vi "(Depricated) Sample Trasfer Base Pressure Mean.vi"(3 "sample length (10)":i32=10, 4 "initialize on the next call":bool, 5 "Baratron 1":dbl format="%0.2f") -> (0 "d":dbl(graph), 1 "mean":dbl format="%0.2f")   [LabVIEW 2015, in "cRIO-Carbondioxide.lvlib" / "cRIO-CO2.lvlib" / "cRIO-CO2.lvclass"]
uses:
  cRIO-CO2.lvclass
  <vilib>/ptbypt/NI_PtbyPt.lvlib
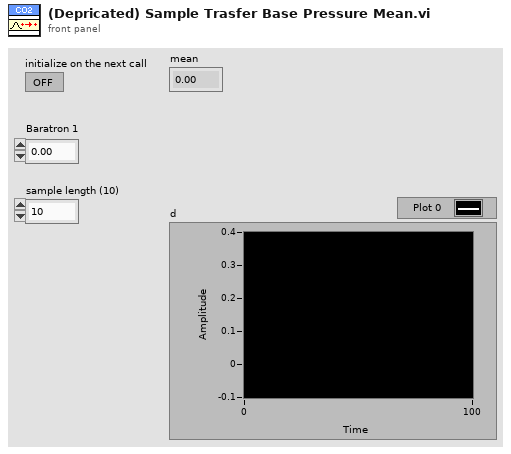
[diagram p1: front panel]
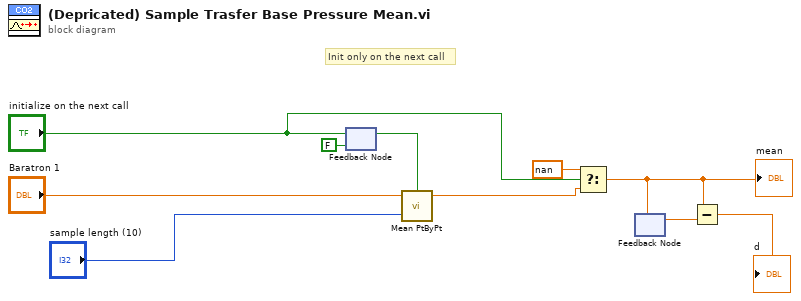
[diagram p0: block diagram]
diagram:
  # "Init only on the next call"
  n1 = feedback-in #1("initialize on the next call") -> ()
  n2 = feedback #1(FALSE ("initialize")) -> (w8:bool)
  n3 = call <vilib>:"Mean PtByPt.vi"("x"="Baratron 1", "sample length"="sample length (10)", "initialize"=w8) -> ("mean"=w1:dbl)  [unwired: 1 in, 1 out]
  n4 = Select(t=nan, s="initialize on the next call", f=w1) -> (s? t:f=w3:dbl)
  "mean" <- w3
  n5 = feedback-in #2(w3) -> ()
  n6 = feedback #2() -> (w4:dbl)  [unwired: 1 in]
  n7 = Subtract(x=w3, y=w4) -> (x-y=→"d":dbl)
